vi "Error Query.vi"(8 "error in (no error)":errorcluster, 11 "VISA resource name":refnum<visa-resource-name>) -> (0 "error out":errorcluster, 1 "Error Message":string, 2 "Error Code":i32[](array[numeric]), 3 "VISA resource name out":refnum<visa-resource-name>)   [LabVIEW 2018, in "Keithley KE22xx Series.lvlib"]
doc: "Queries the instrument for any errors in the instrument's error queue. It will continue to read errors until all errors have been read from the instrument. Any errors will be returned in the <B>error out</B> control.\n\n<B>Note:</B>\nThis VI is called automatically by most driver VIs so it is not usually necessary to call this in an application."
uses:
  Keithley KE22xx Series.lvlib
panel:
  # "© 2012 Keithley Instruments, Inc. ALL RIGHTS RESERVED"
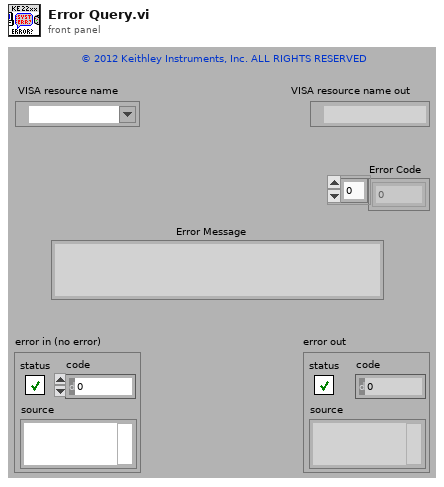
[diagram p1: front panel]
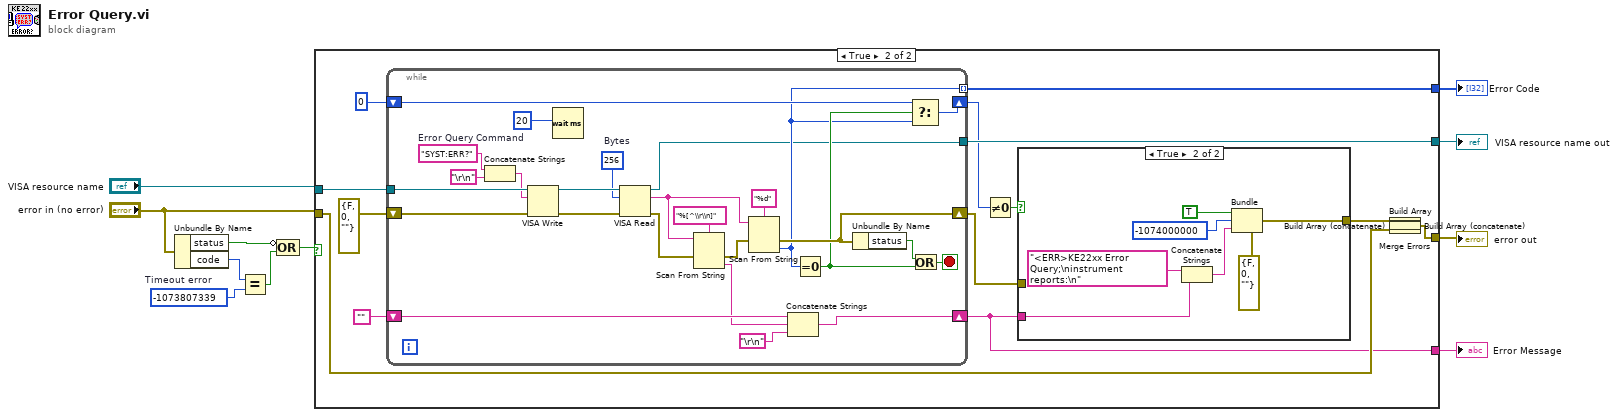
[diagram p0: block diagram]
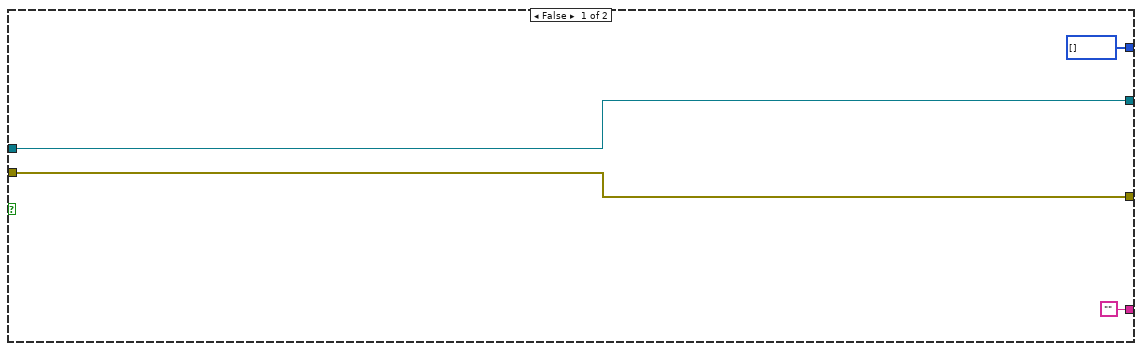
[diagram p2: hidden frame]
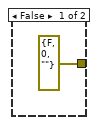
[diagram p3: hidden frame]
diagram:
  w10 = -1073807339  # Timeout error
  n1 = Unbundle By Name("error in (no error)") -> ("status"=w11:bool, "code"=w8:i32)
  n2 = Equal?(x=w8, y=w10) -> (x = y?=w9:bool)
  n3 = Compound Arithmetic op=OR(invert w11, w9) -> (w7:bool)
  n4 = case shown="True" w7 {
    tunnel: [w15 w31] -> w2
    tunnel: "VISA resource name" -> [w15 w30]
    tunnel: "error in (no error)" -> [w14 w24]
    tunnel: [w14 w28] -> w3
    tunnel: ["" w21] -> w4
    tunnel: [i32[] [] w20] -> w1
    frame False {
    }
    frame True {
      n5 = while {
        tunnel: [w43] -> w20 mode=indexing
        shift-left: errorcluster {"status"=FALSE, "code"=0, "source"=""} ("error in (no error)") -> [w48]
        shift-right: [w47] -> w19
        shift-left: 0 -> [w50]
        shift-right: [w49] -> w22
        shift-left: "" -> [w53]
        shift-right: [w51] -> w21
        tunnel: w30 -> [w57]
        tunnel: [w41] -> w31
        stop <- w55 stop-if-true
        w40 = u32 256  # Bytes
        w37 = "SYST:ERR?"  # Error Query Command
        n6 = Concatenate Strings(w37, "\r\n") -> (w36:string)
        n7 = VISA Write(VISA resource name=w57, write buffer=w36, error in (no error)=w48) -> (VISA resource name out=w42:refnum<visa-resource-name>, error out=w34:errorcluster)  [unwired: 1 out]
        n8 = Wait (ms)(milliseconds to wait=u32 20) -> ()  [unwired: 1 out]
        n9 = VISA Read(VISA resource name=w42, byte count=w40, error in (no error)=w34) -> (VISA resource name out=w41:refnum<visa-resource-name>, read buffer=w38:string, error out=w39:errorcluster)  [unwired: 1 out]
        n10 = Scan From String(format string="%[^\\r\\n]", input string=w38, error in=w39) -> (error out=w46:errorcluster, output 1=w32:string)  [unwired: 1 in, 3 out]
        n11 = Scan From String(format string="%d", input string=w38, error in=w46) -> (error out=w47:errorcluster, output 1=w43:i32)  [unwired: 1 in, 3 out]
        n12 = Concatenate Strings(w53, w32, "\r\n") -> (w51:string)
        n13 = Equal To 0?(x=w43) -> (x = 0?=w44:bool)
        n14 = Unbundle By Name(w47) -> ("status"=w45:bool)
        n15 = Select(t=w50, s=w44, f=w43) -> (s? t:f=w49:i32)
        n16 = Or(x=w45, y=w44) -> (x .or. y?=w55:bool)
      }
      n17 = Not Equal To 0?(x=w22) -> (x != 0?=w26:bool)
      n18 = case shown="True" w26 {
        tunnel: w21 -> [_ w61]
        tunnel: [errorcluster {"status"=FALSE, "code"=0, "source"=""} ("error out") w60] -> w25
        tunnel: w19 -> [_ _]
        frame False {
        }
        frame True {
          n19 = Concatenate Strings("<ERR>KE22xx Error Query;\ninstrument reports:\n" ("Source"), w61) -> (w62:string)
          n20 = Bundle(cluster=errorcluster {"status"=FALSE, "code"=0, "source"=""} ("error out"), "status"=TRUE ("Status"), "code"=-1074000000 ("Code"), "source"=w62) -> (w60:errorcluster)
        }
      }
      n21 = Build Array(w25, w24) -> (w18:errorcluster[])
      n22 = Build Array (concatenate)(w18) -> (w17:errorcluster[])
      n23 = Build Array (concatenate)(w17) -> (w16:errorcluster[])
      n24 = Merge Errors(w16) -> (w28:errorcluster)
    }
  }
  "VISA resource name out" <- w2
  "error out" <- w3
  "Error Message" <- w4
  "Error Code" <- w1
